vi "testCQTDDS.vi"   [LabVIEW 2009]
uses:
  C:/Users/Administrator/Desktop/Crete/DDS/DDS-Control-a8929c3/CQTAD9958/bin/Debug/CQTAD9958.dll
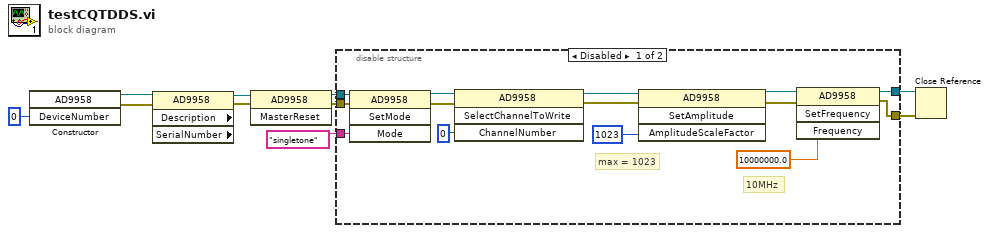
[diagram p0: block diagram]
diagram:
  n1 = constructor class="AD9958"("DeviceNumber"=0) -> (reference out=w9:refnum<k24>, error out=w8:errorcluster)  [unwired: 3 in, 2 out]
  n2 = property class="AD9958" props=["Description", "SerialNumber"](reference=w9, error in=w8) -> (reference out=w7:refnum<k24>, error out=w6:errorcluster)  [unwired: 2 out]
  n3 = invoke class="AD9958" method="MasterReset"(reference=w7, error in=w6) -> (reference out=w5:refnum<k24>, error out=w4:errorcluster)  [unwired: 1 in, 1 out]
  n4 = disable-structure shown="Disabled" {
    disable-tunnel: w5 -> [w24 w26]
    disable-tunnel: w4 -> [w14 w25]
    disable-tunnel: "singletone" -> [w13 _]
    disable-tunnel: [w12 w26] -> w2
    disable-tunnel: [w11 w25] -> w1
    frame #0 {
      # "max = 1023"
      # "10MHz"
      n5 = invoke class="AD9958" method="SetMode"(reference=w24, error in=w14, "Mode"=w13) -> (reference out=w16:refnum<k24>, error out=w15:errorcluster)  [unwired: 1 in, 2 out]
      n6 = invoke class="AD9958" method="SelectChannelToWrite"(reference=w16, error in=w15, "ChannelNumber"=0) -> (reference out=w22:refnum<k24>, error out=w21:errorcluster)  [unwired: 1 in, 2 out]
      n7 = invoke class="AD9958" method="SetAmplitude"(reference=w22, error in=w21, "AmplitudeScaleFactor"=1023) -> (reference out=w19:refnum<k24>, error out=w18:errorcluster)  [unwired: 1 in, 2 out]
      n8 = invoke class="AD9958" method="SetFrequency"(reference=w19, error in=w18, "Frequency"=10000000.0) -> (reference out=w12:refnum<k24>, error out=w11:errorcluster)  [unwired: 1 in, 2 out]
    }
    frame #1 {
    }
  }
  n9 = Close Reference(reference=w2, error in (no error)=w1) -> ()  [unwired: 1 out]
